vi "Starting.vi"(6 "Refs":refnum<class "Refs.lvclass">, 7 "Actor in":refnum<class "Actor.lvclass">, 9 "Actor Ref":refnum<vi>, 10 "Spawn":refnum<class "Spawn.lvclass">) -> (0 "Error out":errorcluster, 5 "Actor out":refnum<class "Actor.lvclass">)   [LabVIEW 2025, in "jettl.lvlib" / "Transport.lvlib" / "Queue.lvlib"]
uses:
  Queue.lvlib
  Refs/Refs.lvclass
  Actor/Actor.lvclass
  Spawn/Spawn/Spawn.lvclass
  jettl.lvlib
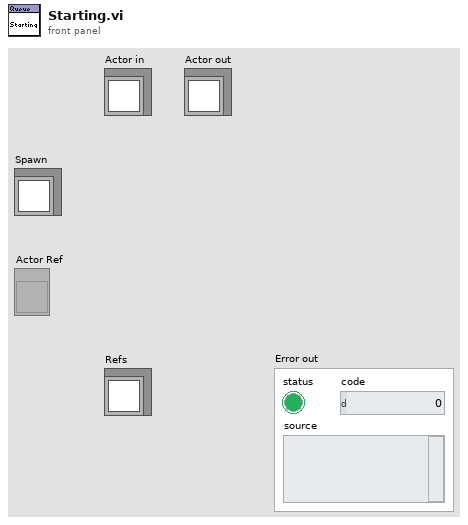
[diagram p1: front panel]
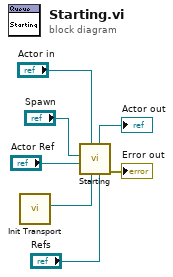
[diagram p0: block diagram]
diagram:
  n1 = call "Init Transport.vi"() -> ("Transport"=w1:refnum<class "Transport.lvclass">)  [unwired: 11 in]
  n2 = call "Starting.vi"("Refs"="Refs", "Transport"=w1, "Actor in"="Actor in", "Actor Ref"="Actor Ref", "Spawn"="Spawn") -> ("Error out"=→"Error out":errorcluster, "Actor out"=→"Actor out":refnum<class "Actor.lvclass">)  [unwired: 5 in]
